vi "Independent Operation.vi"() -> ()   [LabVIEW 2012]
panel:
  in  "Loop 2 stop":bool
  out "Loop 2 Chart":dbl(graph)
  in  "Loop 2 speed":dbl(knob) scale=0.0..1000.0
  in  "Loop 1 speed":dbl(knob) scale=0.0..1000.0
  out "Loop 1 Chart":dbl(graph)
  in  "Loop 1 stop":bool
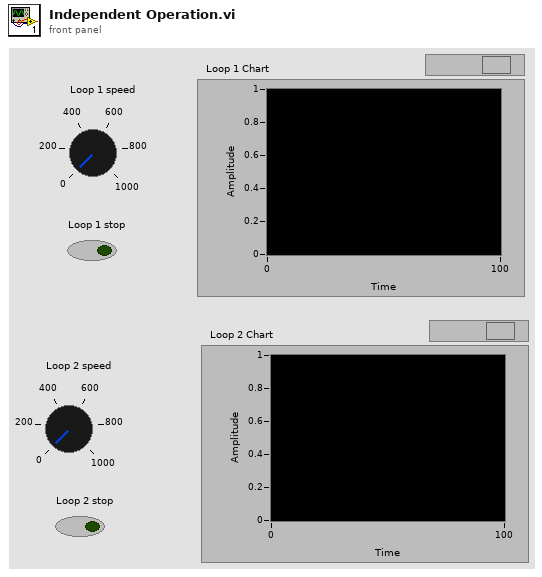
[diagram p1: front panel]
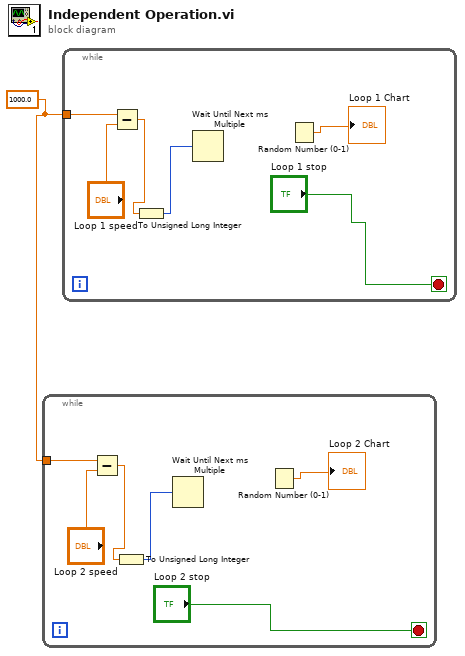
[diagram p0: block diagram]
diagram:
  w1 = 1000.0 ("x")
  n1 = while {
    tunnel: w1 -> [w3]
    stop <- "Loop 2 stop" stop-if-true
    n2 = Subtract(x=w3, y="Loop 2 speed") -> (x-y=w5:dbl)
    n3 = To Unsigned Long Integer(number=w5) -> (unsigned 32bit integer=w6:u32)
    n4 = Wait Until Next ms Multiple(millisecond multiple=w6) -> ()  [unwired: 1 out]
    n5 = Random Number (0-1)() -> (number: 0 to 1=→"Loop 2 Chart":dbl)
  }
  n6 = while {
    tunnel: w1 -> [w9]
    stop <- "Loop 1 stop" stop-if-true
    n7 = Subtract(x=w9, y="Loop 1 speed") -> (x-y=w11:dbl)
    n8 = To Unsigned Long Integer(number=w11) -> (unsigned 32bit integer=w12:u32)
    n9 = Wait Until Next ms Multiple(millisecond multiple=w12) -> ()  [unwired: 1 out]
    n10 = Random Number (0-1)() -> (number: 0 to 1=→"Loop 1 Chart":dbl)
  }
